vi "Servo MSMT GSM Configure Fetch Step.vi"(8 "error in (no error)":errorcluster, 11 "Servo MSMT in":refnum<class "Servo MSMT.lvclass">) -> (0 "error out":errorcluster, 3 "Servo MSMT out":refnum<class "Servo MSMT.lvclass">)   [LabVIEW 2018, in "Servo MSMT.lvlib" / "Servo MSMT.lvclass"]
uses:
  Servo MSMT.lvclass
  C:/Sequence Automation/Plugins/Measurement Interface.lvlibp/Measurement Interface.lvclass
  Plugins/Measurement Interface.lvlibp/Private Methods/Measurement Name/Read Measurement Name.vi
  Plugins/Measurement Interface.lvlibp/Private Methods/Engine Reference/Read Engine Reference.vi
  Plugins/Measurement Interface.lvlibp/Public Methods/Sequence Reference/Read Sequence Reference.vi
  Plugins/TestStand API Tools (TSAT).lvlibp/Step Actions/TSAT Step Actions.lvlib
  Plugins/TestStand API Tools (TSAT).lvlibp/Sequence Actions/TSAT Sequence Actions.lvlib
  Plugins/Measurement Interface.lvlibp/Measurement Interface.lvclass
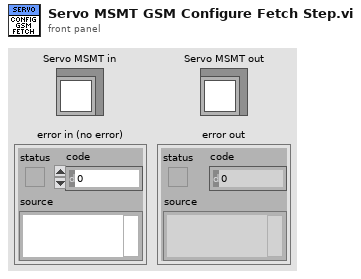
[diagram p1: front panel]
types:
  T1 = typedef "TestStand API Tools (TSAT).lvlibp/TSAT Evaluation Actions.lvlib/TSAT Evaluation.ctl" = cluster{"Test Name":string, "Pin":string, "Units":string, "SI Scaling":T2, "Test Number":i32, "Published Data Id":string, "Low Limit":dbl, "High Limit":dbl, "Export Data Location":string, "Software Bin":i64, "Evaluation Type":T3, "Test Data Source":string}
  T2 = typedef "TestStand API Tools (TSAT).lvlibp/TSAT Evaluation Actions.lvlib/TSAT Eval SI Unit Scaling.ctl" = i16
  T3 = typedef "TestStand API Tools (TSAT).lvlibp/TSAT Evaluation Actions.lvlib/TSAT Evaluation Type.ctl" = enum16{"Numeric Limit", "Pass/Fail", "None"}
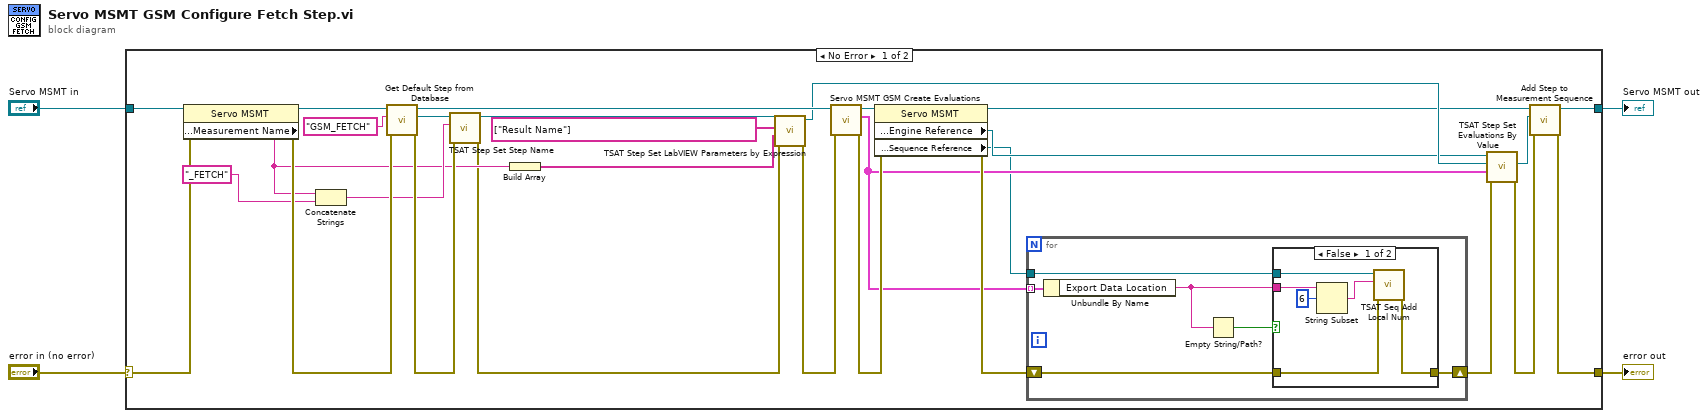
[diagram p0: block diagram]
diagram:
  n1 = case shown="No Error" "error in (no error)" {
    selector: "error in (no error)" -> [w28 w48]
    tunnel: [w19 w48] -> w3
    tunnel: [w18 w47] -> w1
    tunnel: "Servo MSMT in" -> [w33 w47]
    frame No Error {
      n2 = property class="Servo MSMT"(reference=w33, error in=w28) -> (reference out=w29:refnum<class "Servo MSMT.lvclass">, error out=w27:errorcluster, "Public Methods:Measurement Name"=w25:string)
      n3 = Concatenate Strings(w25, "_FETCH" ("string")) -> (w26:string)
      n4 = call "Get Default Step from Database.vi"("error in (no error)"=w27, "Default Step"="GSM_FETCH", "Measurement Interface in"=w29) -> ("error out"=w31:errorcluster, "Cloned Step"=w32:refnum<k7>, "Measurement Interface out"=w20:refnum<class "Servo MSMT.lvclass">)  [unwired: 6 in]
      n5 = call "TSAT Step Set Step Name.vi"("Error In"=w31, "Name"=w26, "Step In"=w32) -> ("Error Out"=w23:errorcluster, "Step Out"=w30:refnum<k7>)  [unwired: 7 in]
      n6 = Build Array(w25) -> (w24:string[])
      n7 = call "TSAT Step Set LabVIEW Parameters by Expression.vi"("Error In"=w23, "Value Expressions"=w24, "Parameters to Set"=string[] ["Result Name"], "Step In"=w30) -> ("Error Out"=w22:errorcluster, "Step Out"=w16:refnum<k7>)  [unwired: 6 in]
      n8 = call "Servo MSMT GSM Create Evaluations.vi"("error in (no error)"=w22, "Servo MSMT in"=w20) -> ("error out"=w15:errorcluster, "GSM Evaluations"=w7:T1[], "Servo MSMT out"=w13:refnum<class "Servo MSMT.lvclass">)  [unwired: 7 in]
      n9 = property class="Servo MSMT"(reference=w13, error in=w15) -> (reference out=w12:refnum<class "Servo MSMT.lvclass">, error out=w8:errorcluster, "Protected Methods:Engine Reference"=w11:refnum<k7>, "Public Methods:Sequence Reference"=w6:refnum<k7>)
      n10 = for {
        tunnel: w7 -> [w39] mode=indexing
        shift-right: [w37] -> w5
        shift-left: w8 -> [w38]
        tunnel: w6 -> [w36]
        n11 = Unbundle By Name(w39) -> ("Export Data Location"=w34:string)
        n12 = Empty String/Path?(string/path=w34) -> (empty?=w35:bool)
        n13 = case shown="False" w35 {
          tunnel: w38 -> [w43 w46]
          tunnel: [w42 w46] -> w37
          tunnel: w36 -> [w41 _]
          tunnel: w34 -> [w40 _]
          frame False {
            n14 = String Subset(string=w40, offset (0)=6) -> (substring=w44:string)  [unwired: 1 in]
            n15 = call "TSAT Seq Add Local Num.vi"("Error In"=w43, "Local Variable Name"=w44, "Sequence In"=w41) -> ("Error Out"=w42:errorcluster)  [unwired: 7 in, 1 out]
          }
          frame True {
          }
        }
      }
      n16 = call "TSAT Step Set Evaluations By Value.vi"("Error In"=w5, "Evaluation Data"=w7, "Step In"=w16, "Engine In"=w11) -> ("Error Out"=w14:errorcluster, "Step Out"=w17:refnum<k7>)  [unwired: 5 in, 1 out]
      n17 = call "Add Step to Measurement Sequence.vi"("error in (no error)"=w14, "Step to Add"=w17, "Measurement Interface in"=w12) -> ("error out"=w19:errorcluster, "Measurement Interface out"=w18:refnum<class "Servo MSMT.lvclass">)  [unwired: 7 in]
    }
    frame Error {
    }
  }
  "error out" <- w3
  "Servo MSMT out" <- w1
